vi "BRig_RT__Case_Exp__storeData__endExp__v3.vi"(0 "input_dataBlock":u16[][](array[numeric]), 1 "input_dataCurrent":u16[](array[numeric]), 2 "input_dataLick":u16[][](array[numeric]), 3 "input_dataLC":u16[](array[numeric]), 4 "input_dataExp":u16[](array[numeric]), 5 "input_dataTrial":u16[][](array[numeric]), 7 "input_dataExp_end":u16[](array[numeric]), 9 "input_dataLC_end":u16[](array[numeric]), 11 "input_dataMTrig":u16[](array[numeric]), 12 "input_dataAnalog":u16[][](array[numeric]), 13 "input_dataAnalog_length":i32) -> (15 "output_True":bool)   [LabVIEW 2014]
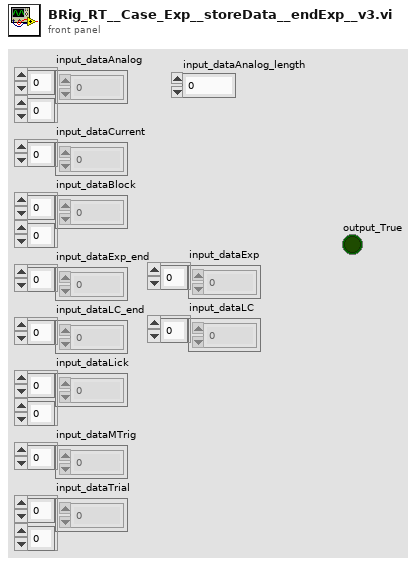
[diagram p1: front panel]
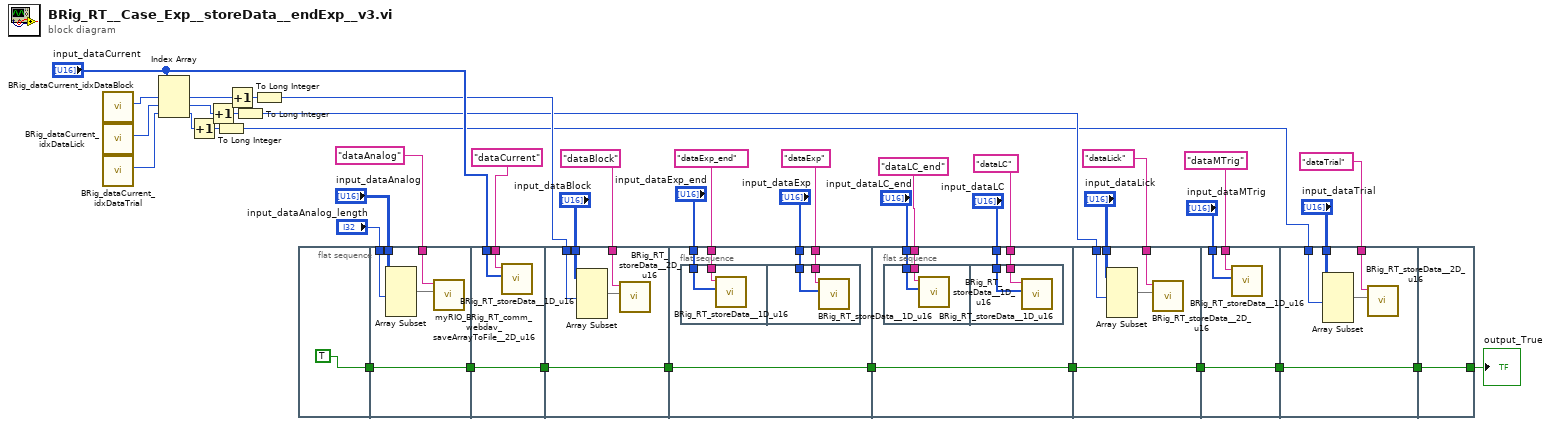
[diagram p0: block diagram]
diagram:
  n1 = call "BRig_dataCurrent_idxDataBlock.vi"() -> ("output_idxDataBlock"=w19:i32)  [unwired: 11 in]
  n2 = call "BRig_dataCurrent_idxDataLick.vi"() -> ("output_idxDataLick"=w18:i32)  [unwired: 11 in]
  n3 = call "BRig_dataCurrent_idxDataTrial.vi"() -> ("output_idxDataTrial"=w17:i32)  [unwired: 11 in]
  n4 = Index Array(array="input_dataCurrent", index #1=w19, index #2=w18, index #3=w17) -> (element #1=w16:u16, element #2=w14:u16, element #3=w11:u16)
  n5 = Increment(x=w11) -> (x+1=w12:u16)
  n6 = Increment(x=w14) -> (x+1=w13:u16)
  n7 = To Long Integer(number=w12) -> (32bit integer=w20:i32)
  n8 = Increment(x=w16) -> (x+1=w15:u16)
  n9 = To Long Integer(number=w13) -> (32bit integer=w26:i32)
  n10 = To Long Integer(number=w15) -> (32bit integer=w37:i32)
  n11 = flat-sequence {
    tunnel: [TRUE] -> w2
    tunnel: "input_dataAnalog_length" -> [w48]
    tunnel: "input_dataAnalog" -> [w47]
    tunnel: "dataAnalog" ("input_filename") -> [w46]
    tunnel: [w45] -> w3
    tunnel: w2 -> [w45]
    tunnel: "dataCurrent" ("input_filename") -> [w52]
    tunnel: "input_dataCurrent" -> [w51]
    tunnel: [w50] -> w4
    tunnel: w3 -> [w50]
    tunnel: "input_dataBlock" -> [w57]
    tunnel: w37 -> [w56]
    tunnel: "dataBlock" ("input_filename") -> [w54]
    tunnel: [w53] -> w5
    tunnel: w4 -> [w53]
    tunnel: "input_dataExp_end" -> [w62]
    tunnel: "dataExp_end" ("input_filename") -> [w61]
    tunnel: "input_dataExp" -> [w60]
    tunnel: "dataExp" ("input_filename") -> [w59]
    tunnel: [w58] -> w6
    tunnel: w5 -> [w58]
    tunnel: "input_dataLC_end" -> [w71]
    tunnel: "dataLC_end" ("input_filename") -> [w70]
    tunnel: "dataLC" ("input_filename") -> [w69]
    tunnel: "input_dataLC" -> [w68]
    tunnel: [w67] -> w7
    tunnel: w6 -> [w67]
    tunnel: "input_dataLick" -> [w80]
    tunnel: w26 -> [w79]
    tunnel: "dataLick" ("input_filename") -> [w77]
    tunnel: [w76] -> w8
    tunnel: w7 -> [w76]
    tunnel: "input_dataMTrig" -> [w83]
    tunnel: "dataMTrig" ("input_filename") -> [w82]
    tunnel: [w81] -> w9
    tunnel: w8 -> [w81]
    tunnel: "input_dataTrial" -> [w88]
    tunnel: "dataTrial" ("input_filename") -> [w86]
    tunnel: w20 -> [w85]
    tunnel: [w84] -> w10
    tunnel: w9 -> [w84]
    tunnel: [w89] -> w1
    tunnel: w10 -> [w89]
    frame #0 {
    }
    frame #1 {
      n12 = Array Subset(array=w47, length (row)=w48) -> (w49:u16[][])  [unwired: 3 in]
      n13 = call "myRIO_BRig_RT_comm_webdav_saveArrayToFile__2D_u16.vi"("Array"=w49, "input_filename"=w46) -> ()  [unwired: 10 in]
    }
    frame #2 {
      n14 = call "BRig_RT_storeData__1D_u16.vi"("Array"=w51, "input_filename"=w52) -> ()  [unwired: 10 in]
    }
    frame #3 {
      n15 = Array Subset(array=w57, length (row)=w56) -> (w55:u16[][])  [unwired: 3 in]
      n16 = call "BRig_RT_storeData__2D_u16.vi"("Array"=w55, "input_filename"=w54) -> ()  [unwired: 10 in]
    }
    frame #4 {
      n17 = flat-sequence {
        tunnel: w62 -> [w64]
        tunnel: w61 -> [w63]
        tunnel: w60 -> [w65]
        tunnel: w59 -> [w66]
        frame #0 {
          n18 = call "BRig_RT_storeData__1D_u16.vi"("Array"=w64, "input_filename"=w63) -> ()  [unwired: 10 in]
        }
        frame #1 {
          n19 = call "BRig_RT_storeData__1D_u16.vi"("Array"=w65, "input_filename"=w66) -> ()  [unwired: 10 in]
        }
      }
    }
    frame #5 {
      n20 = flat-sequence {
        tunnel: w71 -> [w73]
        tunnel: w70 -> [w72]
        tunnel: w69 -> [w75]
        tunnel: w68 -> [w74]
        frame #0 {
          n21 = call "BRig_RT_storeData__1D_u16.vi"("Array"=w73, "input_filename"=w72) -> ()  [unwired: 10 in]
        }
        frame #1 {
          n22 = call "BRig_RT_storeData__1D_u16.vi"("Array"=w74, "input_filename"=w75) -> ()  [unwired: 10 in]
        }
      }
    }
    frame #6 {
      n23 = Array Subset(array=w80, length (row)=w79) -> (w78:u16[][])  [unwired: 3 in]
      n24 = call "BRig_RT_storeData__2D_u16.vi"("Array"=w78, "input_filename"=w77) -> ()  [unwired: 10 in]
    }
    frame #7 {
      n25 = call "BRig_RT_storeData__1D_u16.vi"("Array"=w83, "input_filename"=w82) -> ()  [unwired: 10 in]
    }
    frame #8 {
      n26 = Array Subset(array=w88, length (row)=w85) -> (w87:u16[][])  [unwired: 3 in]
      n27 = call "BRig_RT_storeData__2D_u16.vi"("Array"=w87, "input_filename"=w86) -> ()  [unwired: 10 in]
    }
    frame #9 {
    }
  }
  "output_True" <- w1
